vi "init opc datasocket connection.vi"(7 "AccessMode (ReadAutoUpdate)":T2(ring), 8 "error in":errorcluster, 9 "use opc":bool, 10 "PLC Path":string, 11 "tag":string) -> (0 "error out":errorcluster, 3 "DataSocket Reference Out":T1 {"OnStatusUpdated" format="%.0x"; "OnDataUpdated" format="%.0x"})   [LabVIEW 2018]
uses:
  <vilib>/Platform/dataskt.llb/DataSocket Reference Type.ctl
  <vilib>/Utility/error.llb/DialogType.ctl
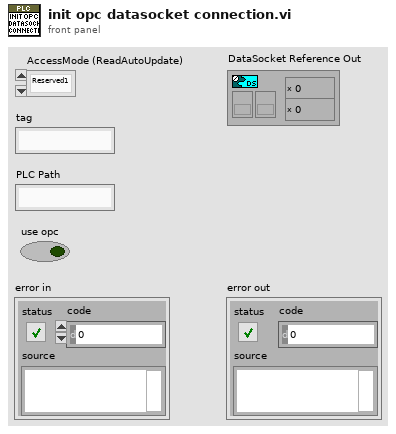
[diagram p1: front panel]
types:
  T1 = typedef "DataSocket Reference Type.ctl" = cluster{"CWDSLib._DCWDataSocket":refnum<k7>, "CWDSLib._DCWData":refnum<k7>, "OnDataUpdated":u32, "OnStatusUpdated":u32}
  T2 = enum32{"Reserved1", "Reserved2", "Read", "ReadAutoUpdate", "Write", "WriteAutoUpdate"}
  T3 = typedef "DialogType.ctl" = u16
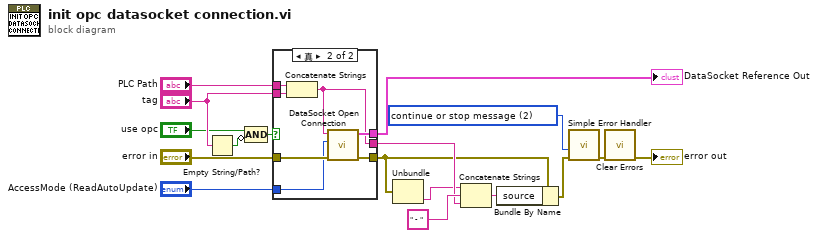
[diagram p0: block diagram]
diagram:
  w8 = T3 2 items=["no dialog", "OK message", "continue or stop message", "OK message + warnings", "continue/stop + warnings"] ("type of dialog (OK msg:1)")
  n1 = Empty String/Path?(string/path="tag") -> (empty?=w11:bool)
  n2 = Compound Arithmetic op=AND("use opc", invert w11) -> (w10:bool)
  n3 = case shown="真" w10 {
    tunnel: "PLC Path" -> [_ w25]
    tunnel: "tag" -> [_ w24]
    tunnel: [_ w23] -> w3
    tunnel: "error in" -> [w18 w22]
    tunnel: [w18 w21] -> w12
    tunnel: "AccessMode (ReadAutoUpdate)" -> [_ w20]
    tunnel: [_ w19] -> w15
    frame False {
    }
    frame True {
      n4 = Concatenate Strings(w25, w24) -> (w19:string)
      n5 = call <vilib>:"DataSocket Open Connection.vi"("error in (no error)"=w22, "AccessMode (ReadAutoUpdate)"=w20, "URL"=w19) -> ("error out"=w21:errorcluster, "DataSocket Reference Out"=w23:T1)  [unwired: 5 in]
    }
  }
  "DataSocket Reference Out" <- w3
  n6 = Unbundle(w12) -> ("source"=w14:string)  [unwired: 2 out]
  n7 = Concatenate Strings(w14, " - " ("string"), w15) -> (w13:string)
  n8 = Bundle By Name(cluster=w12, "source"=w13) -> (w16:errorcluster)
  n9 = call <vilib>:"Simple Error Handler.vi"("type of dialog (OK msg:1)"=w8, "error in (no error)"=w16) -> ("error out"=w6:errorcluster)  [unwired: 3 in, 4 out]
  n10 = call <vilib>:"Clear Errors.vi"("error in (no error)"=w6) -> ("error out"=→"error out":errorcluster)  [unwired: 5 in, 1 out]
